vi "Set Trigger.vi"(8 "error in (no error)":errorcluster, 10 "Trigger Settings":T1={"Edge:"=0, "Level"=0.0, "Source"=0, "trigger coupling"=1, "Holdoff"=0.0, "Delay"=0.0, "Trigger Modifier"=enum."Auto Trigger", "Trigger Type"=enum."Analog Edge"} {"trigger coupling" items=["AC", "DC", "HF Reject", "LF Reject", "AC Plus HF Reject"]; "Source" items=["Channel_1", "Channel_2", "Channel_3", "Channel_4", "Channel_5", "Channel_6", "Channel_7", "Channel_8"]; "Edge:" items=["Rising Edge", "Falling Edge"]}, 11 "5105 in":refnum<class "5105.lvclass">) -> (0 "error out":errorcluster, 3 "5105 out":refnum<class "5105.lvclass">)   [LabVIEW 2019, in "5105.lvlib" / "5105.lvclass"]
uses:
  5105.lvclass
  builds/Instruments/Oscilloscope.lvlibp/Custom Controls/Trigger Settings.ctl
  builds/Instruments/Oscilloscope.lvlibp/Custom Controls/Edge Select.ctl
  builds/Instruments/Oscilloscope.lvlibp/Custom Controls/Channel List.ctl
  builds/Instruments/Oscilloscope.lvlibp/Custom Controls/Trigger Coupling.ctl
  builds/Instruments/Oscilloscope.lvlibp/Custom Controls/Trigger Modifier.ctl
  builds/Instruments/Oscilloscope.lvlibp/Custom Controls/Trigger Type.ctl
  builds/Instruments/Oscilloscope.lvlibp/Oscilloscope.lvclass
  C:/Users/Public/Documents/Development/builds/Instruments/Oscilloscope.lvlibp/Oscilloscope.lvclass
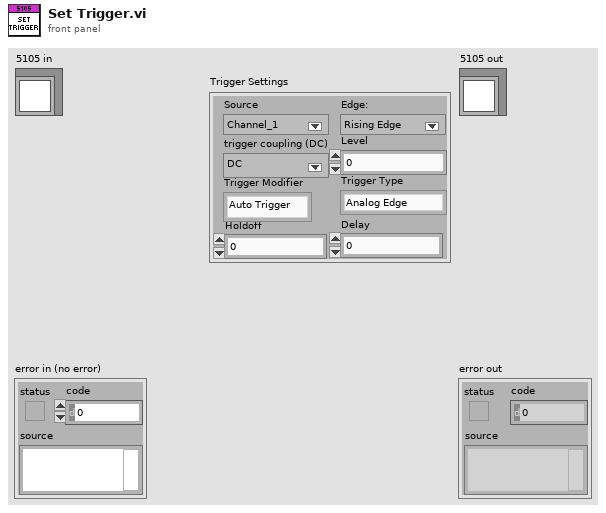
[diagram p1: front panel]
types:
  T1 = typedef "Oscilloscope.lvlibp/Oscilloscope.lvclass/Trigger Settings.ctl" = cluster{"Edge:":T2, "Level":dbl, "Source":T3, "trigger coupling":T4, "Holdoff":dbl, "Delay":dbl, "Trigger Modifier":T5, "Trigger Type":T6}
  T2 = typedef "Oscilloscope.lvlibp/Oscilloscope.lvclass/Edge Select.ctl" = u16
  T3 = typedef "Oscilloscope.lvlibp/Oscilloscope.lvclass/Channel List.ctl" = u16
  T4 = typedef "Oscilloscope.lvlibp/Oscilloscope.lvclass/Trigger Coupling.ctl" = u16
  T5 = typedef "Oscilloscope.lvlibp/Oscilloscope.lvclass/Trigger Modifier.ctl" = enum16{"Invalid_Setting", "None", "Auto Trigger"}
  T6 = typedef "Oscilloscope.lvlibp/Oscilloscope.lvclass/Trigger Type.ctl" = enum16{"Immediate", "Analog Edge", "Digital", "Window", "Hysteresis"}
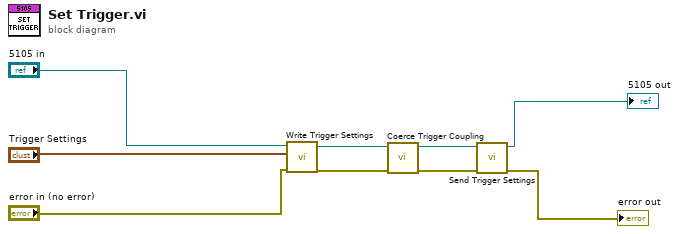
[diagram p0: block diagram]
diagram:
  n1 = call "Write Trigger Settings.vi"("error in"="error in (no error)", "Trigger Settings"="Trigger Settings", "Oscilloscope in"="5105 in") -> ("error out"=w6:errorcluster, "Oscilloscope out"=w7:refnum<class "5105.lvclass">)  [unwired: 7 in]
  n2 = call "Coerce Trigger Coupling.vi"("error in (no error)"=w6, "5105 in"=w7) -> ("error out"=w3:errorcluster, "5105 out"=w4:refnum<class "5105.lvclass">)  [unwired: 8 in]
  n3 = call-dynamic "Send Trigger Settings.vi"("error in (no error)"=w3, "5105 in"=w4) -> ("error out"=→"error out":errorcluster, "5105 out"=→"5105 out":refnum<class "5105.lvclass">)  [unwired: 8 in]
